vi "SV Remove Delays (N,N) from Waveforms (N Ch) (DBL).vi"(7 "reset":bool, 8 "error in (no error)":errorcluster, 9 "path-dependent analog delays [s]":dbl[](array[numeric]) format="%.2p", 10 "channel-dependent digital delays [samples]":dbl[](array[numeric]) min=0.0 format="%.1f", 11 "scaled signals":waveform(dbl)[](array[waveform])) -> (0 "error out":errorcluster, 1 "residual delays [s]":dbl[](array[numeric]) format="%.2p", 2 "aligned signals length":i32, 3 "aligned signals":waveform(dbl)[](array[waveform]))   [LabVIEW 2017]
doc: "Use this VI to align waveforms for channels with propagation delay. For each channel, signal delay is added such that all signals have the same (maximum) delay. This common delay is then removed from all signals. This VI maintains a FIFO for each channel to keep the signals aligned with subsequent calls to the VI. The output waveforms will all have the same length. This VI may output waveforms with a different length on reset=TRUE or first call than in subsequent calls."
uses:
  <vilib>/addons/_NISVFA/_Shared subVIs/Common/svc_Check for Waveform Parameter Continuity (no state).vi
  <vilib>/addons/_NISVFA/_Shared subVIs/Common/svc_Get SV Channel Info.vi
  <vilib>/addons/_NISVFA/_Shared subVIs/Common/svc_Engineering Units to Unit Label.vi
  <vilib>/addons/_NISVFA/_Shared subVIs/Common/svc_Unit Label to Engineering Units.vi
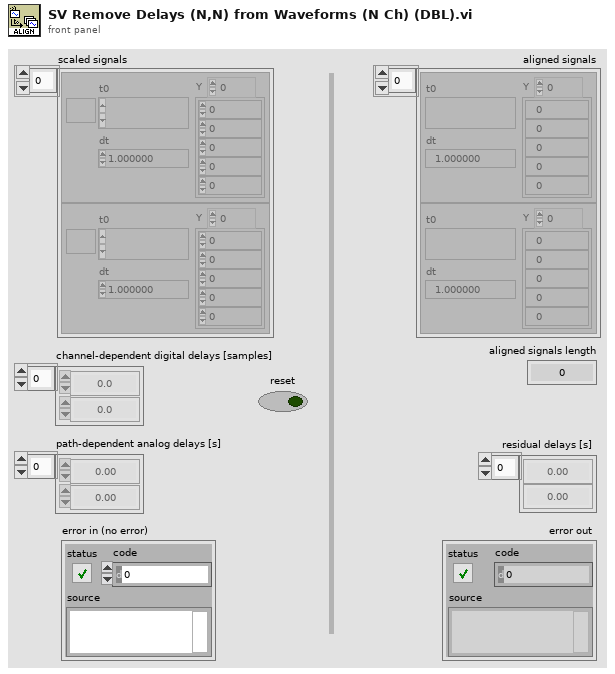
[diagram p1: front panel]
types:
  T1 = cluster{"dt equal":bool, "array length equal":bool, "number channels change":bool}
  T2 = cluster{"dt":bool, "t0 continuity":bool, "array length":bool, "channel info":bool, "name":bool}
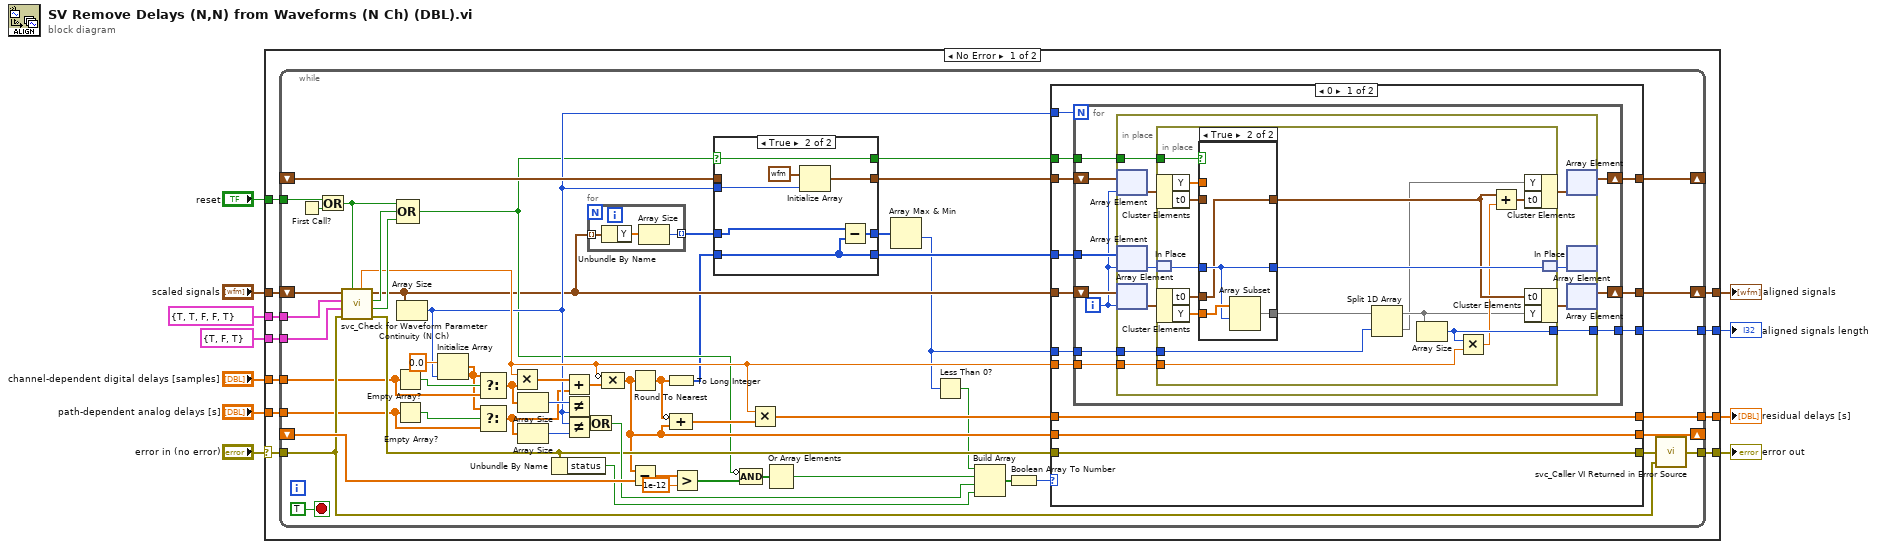
[diagram p0: block diagram]
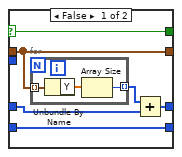
[diagram p2: hidden frame]
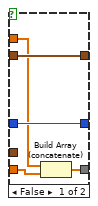
[diagram p3: hidden frame]
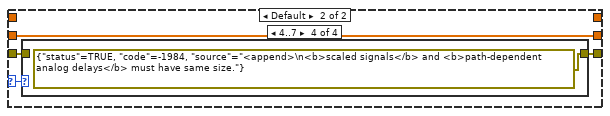
[diagram p4: hidden frame]
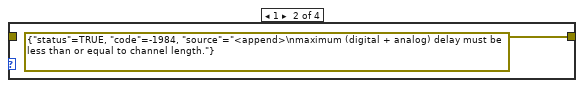
[diagram p6: hidden frame]
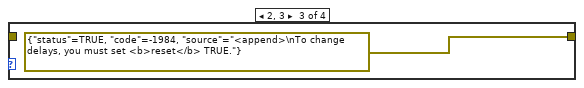
[diagram p7: hidden frame]
diagram:
  n1 = case shown="No Error" "error in (no error)" {
    selector: "error in (no error)" -> [w15 w167]
    tunnel: "scaled signals" -> [w22 _]
    tunnel: "channel-dependent digital delays [samples]" -> [w14 _]
    tunnel: "path-dependent analog delays [s]" -> [w12 _]
    tunnel: [w17 _] -> w7
    tunnel: [w19 _] -> w6
    tunnel: "reset" -> [w16 _]
    tunnel: T2 {"dt"=TRUE, "t0 continuity"=TRUE, "array length"=FALSE, "channel info"=FALSE, "name"=TRUE} ("checks for channel parameter change") -> [w21 _]
    tunnel: T1 {"dt equal"=TRUE, "array length equal"=FALSE, "number channels change"=TRUE} ("checks for multichannel parameters") -> [w20 _]
    tunnel: [w18 w167] -> w2
    tunnel: [w13 _] -> w1
    frame No Error {
      n2 = while {
        tunnel: w21 -> [w80]
        tunnel: w20 -> [w79]
        tunnel: [w77] -> w19
        tunnel: [w52] -> w18
        tunnel: w16 -> [w72]
        tunnel: w15 -> [w50]
        tunnel: w14 -> [w41]
        tunnel: [w69] -> w13
        tunnel: w12 -> [w36]
        shift-right: [w65] -> _
        shift-left: _ -> [w63]
        shift-right: [w75] -> w17
        shift-left: w22 -> [w81]
        shift-right: [w48] -> _
        shift-left: _ -> [w47]
        stop <- TRUE stop-if-true
        n3 = First Call?() -> (First Call?: T/F=w31:bool)
        n4 = Or(x=w72, y=w31) -> (x .or. y?=w71:bool)
        n5 = call <vilib>:"svc_Check for Waveform Parameter Continuity (N Ch).vi"("restart averaging (F)"=w71, "error in (no error)"=w50, "checks for multichannel parameters"=w79, "checks for channel parameter change"=w80, "scaled signal(s)"=w81) -> ("error out"=w53:errorcluster, "multichannel parameter changed"=w73:bool, "waveform parameter changed"=w74:bool, "dup scaled signal(s)"=w29:waveform(dbl)[], "dt"=w49:dbl)  [unwired: 2 out]
        n6 = Empty Array?(array=w41) -> (empty?=w39:bool)
        n7 = Empty Array?(array=w36) -> (empty?=w37:bool)
        n8 = Compound Arithmetic op=OR(w71, w74, w73) -> (w30:bool)
        n9 = Array Size(array=w29) -> (size(s)=w38:i32)
        n10 = Initialize Array(0.0 ("element"), w38) -> (w35:dbl[])
        n11 = Select(t=w35, s=w39, f=w41) -> (s? t:f=w40:dbl[])
        n12 = Select(t=w35, s=w37, f=w36) -> (s? t:f=w34:dbl[])
        n13 = Multiply(x=w49, y=w40) -> (x*y=w67:dbl[])
        n14 = Array Size(array=w40) -> (size(s)=w43:i32)
        n15 = Array Size(array=w34) -> (size(s)=w68:i32)
        n16 = Unbundle By Name(w53) -> ("status"=w56:bool)
        n17 = Add(x=w67, y=w34) -> (x+y=w66:dbl[])
        n18 = Not Equal?(x=w43, y=w38) -> (x != y?=w33:bool)
        n19 = Not Equal?(x=w38, y=w68) -> (x != y?=w32:bool)
        n20 = Or(x=w33, y=w32) -> (x .or. y?=w57:bool)
        n21 = for {
          tunnel: w29 -> [w84] mode=indexing
          tunnel: [w82] -> w26 mode=indexing
          n22 = Unbundle By Name(w84) -> ("Y"=w83:dbl[])
          n23 = Array Size(array=w83) -> (size(s)=w82:i32)
        }
        n24 = Compound Arithmetic op=MULTIPLY(invert w49, w66) -> (w44:dbl[])
        n25 = Round To Nearest(number=w44) -> (nearest integer value=w70:dbl[])
        n26 = Subtract(x=w44, y=w63) -> (x-y=w61:dbl[])
        n27 = To Long Integer(number=w70) -> (32bit integer=w28:i32[])
        n28 = Compound Arithmetic op=ADD(invert w70, w44) -> (w78:dbl[])
        n29 = Greater?(x=w61, y=1e-12) -> (0:w62:bool[])
        n30 = case shown="True" w30 {
          selector: w30 -> [w90 w97]
          tunnel: [w88 w100] -> w46
          tunnel: w38 -> [_ w99]
          tunnel: w47 -> [w88 _]
          tunnel: [w90 w97] -> w45
          tunnel: w28 -> [w89 w95]
          tunnel: [w89 w95] -> w27
          tunnel: [w85 w94] -> w24
          tunnel: w26 -> [w86 w96]
          frame False {
            n31 = for {
              tunnel: w88 -> [w93] mode=indexing
              tunnel: [w91] -> w87 mode=indexing
              n32 = Unbundle By Name(w93) -> ("Y"=w92:dbl[])
              n33 = Array Size(array=w92) -> (size(s)=w91:i32)
            }
            n34 = Add(x=w87, y=w86) -> (x+y=w85:i32[])
          }
          frame True {
            n35 = Initialize Array(waveform(dbl) {"t0"=timestamp(0 s since 1904-01-01), "dt"=1.0, "Y"=[]} ("Scaled signal 2"), w99) -> (w100:waveform(dbl)[])
            n36 = Subtract(x=w96, y=w95) -> (x-y=w94:i32[])
          }
        }
        n37 = Compound Arithmetic op=AND(invert w30, w62) -> (w59:bool[])
        n38 = Multiply(x=w49, y=w78) -> (x*y=w76:dbl[])
        n39 = Or Array Elements(Boolean array=w59) -> (logical OR=w58:bool)
        n40 = Array Max & Min(array=w24) -> (min value=w23:i32)  [unwired: 3 out]
        n41 = Less Than 0?(x=w23) -> (x < 0?=w25:bool)
        n42 = Build Array(w25, w58, w57, w56) -> (w54:bool[])
        n43 = Boolean Array To Number(Boolean array=w54) -> (number=w55:u32)
        n44 = case shown="0" w55 {
          selector: w55 -> [_ w161]
          tunnel: w29 -> [w113 _]
          tunnel: [w111 _] -> w77
          tunnel: w76 -> [w111 _]
          tunnel: [w104 w160] -> w51
          tunnel: [w112 _] -> w75
          tunnel: w23 -> [w108 _]
          tunnel: w27 -> [w110 _]
          tunnel: w45 -> [w109 _]
          tunnel: [w107 _] -> w69
          tunnel: w49 -> [w106 _]
          tunnel: [w105 w162] -> w65
          tunnel: w44 -> [w105 w162]
          tunnel: w53 -> [w104 w159]
          tunnel: w46 -> [w103 _]
          tunnel: [w102 _] -> w48
          tunnel: w38 -> [w101 _]
          frame 0 {
            n45 = for {
              N: w101 -> [_]
              shift-right: [w120] -> w112
              shift-left: w113 -> [w122]
              shift-right: [w121] -> w102
              shift-left: w103 -> [w114]
              tunnel: w109 -> [w115]
              tunnel: w108 -> [w118]
              tunnel: [w117] -> w107
              tunnel: w106 -> [w116]
              tunnel: w110 -> [w123]
              i -> [w119]
              n46 = in-place {
                in-place-border: w115 -> [w127]
                in-place-border: w118 -> [w126]
                in-place-border: [w125] -> w117
                in-place-border: w116 -> [w124]
                n47 = in-place-array #1(w114, w119) -> (w131:waveform(dbl))
                n48 = in-place-array #2(w123, w119) -> (w133:i32)
                n49 = in-place-array #3(w122, w119) -> (w128:waveform(dbl))
                n50 = in-place {
                  in-place-border: w127 -> [w149]
                  in-place-border: w126 -> [w134]
                  in-place-border: [w143] -> w125
                  in-place-border: w124 -> [w138]
                  n51 = in-place-cluster #4(w131) -> ("Y"=w147:dbl[], "t0"=w140:timestamp)
                  n52 = in-place-match #5(w133) -> (w146:i32)
                  n53 = in-place-cluster #6(w128) -> ("t0"=w144:timestamp, "Y"=w148:dbl[])
                  n54 = case shown="True" w149 {
                    tunnel: w148 -> [w151 w158]
                    tunnel: w147 -> [w152 _]
                    tunnel: [w150 w155] -> w137
                    tunnel: w146 -> [w154 w157]
                    tunnel: [w154 w157] -> w145
                    tunnel: [w153 w156] -> w142
                    tunnel: w144 -> [_ w156]
                    tunnel: w140 -> [w153 _]
                    frame False {
                      n55 = Build Array (concatenate)(w152, w151) -> (w150:dbl[])
                    }
                    frame True {
                      n56 = Array Subset(array=w158, index=w157) -> (w155:dbl[])  [unwired: 1 in]
                    }
                  }
                  n57 = Split 1D Array(array=w137, index=w134) -> (first subarray=w136:dbl[], second subarray=w135:dbl[])
                  n58 = Array Size(array=w136) -> (size(s)=w143:i32)
                  n59 = Multiply(x=w143, y=w138) -> (x*y=w141:dbl)
                  n60 = Add(x=w142, y=w141) -> (x+y=w139:timestamp)
                  n61 = in-place-cluster #4("Y"=w135, "t0"=w139) -> (w130:waveform(dbl))
                  n62 = in-place-cluster #6("t0"=w142, "Y"=w136) -> (w129:waveform(dbl))
                  n63 = in-place-match #5(w145) -> (w132:i32)
                }
                n64 = in-place-array #1(w130) -> (w121:waveform(dbl)[])  [unwired: 1 out]
                n65 = in-place-array #2(w132) -> ()  [unwired: 2 out]
                n66 = in-place-array #3(w129) -> (w120:waveform(dbl)[])  [unwired: 1 out]
              }
            }
          }
          frame Default {
            n67 = case shown="4..7" w161 {
              tunnel: [w163 errorcluster {"status"=TRUE, "code"=-1984, "source"="<append>\nmaximum (digital + analog) delay must be less than or equal to channel length."} ("error out") errorcluster {"status"=TRUE, "code"=-1984, "source"="<append>\nTo change delays, you must set <b>reset</b> TRUE."} ("error out") errorcluster {"status"=TRUE, "code"=-1984, "source"="<append>\n<b>scaled signals</b> and <b>path-dependent analog delays</b> must have same size."} ("error out")] -> w160
              tunnel: w159 -> [w163 _ _ _]
              frame 8.., Default {
              }
              frame 1 {
              }
              frame 2, 3 {
              }
              frame 4..7 {
              }
            }
          }
        }
        n68 = call <vilib>:"svc_Caller VI Returned in Error Source.vi"("warning input to caller"=w50, "error in (no error)"=w51) -> ("error out"=w52:errorcluster)  [unwired: 3 in]
      }
    }
    frame Error {
    }
  }
  "aligned signals" <- w7
  "error out" <- w2
  "residual delays [s]" <- w6
  "aligned signals length" <- w1
